vi "Get Map.vi"(8 "error in (no error)":errorcluster, 10 "URL":string) -> (0 "error out":errorcluster, 2 "Body":string)   [LabVIEW 2012]
doc: "Requests the given URL and returns the body of the request."
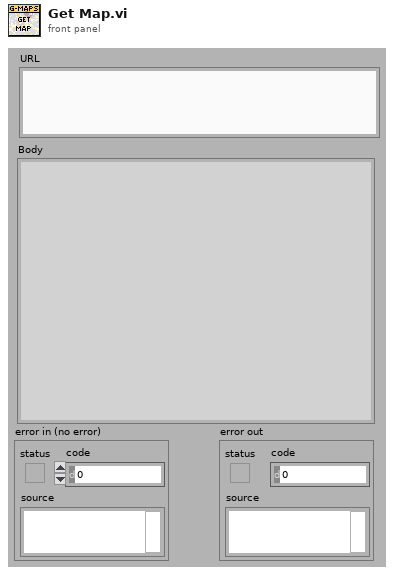
[diagram p1: front panel]
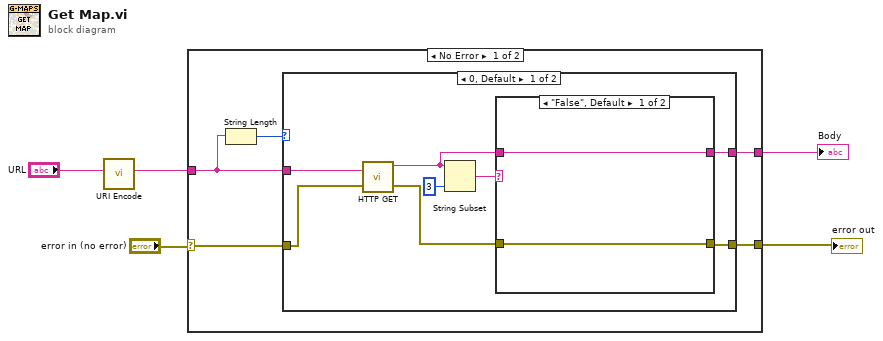
[diagram p0: block diagram]
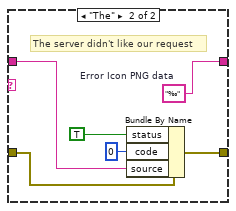
[diagram p2: hidden frame]
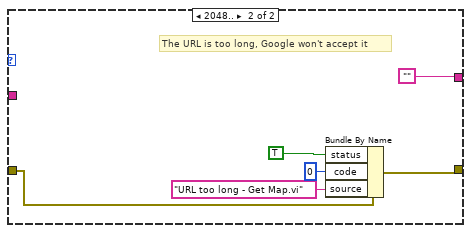
[diagram p3: hidden frame]
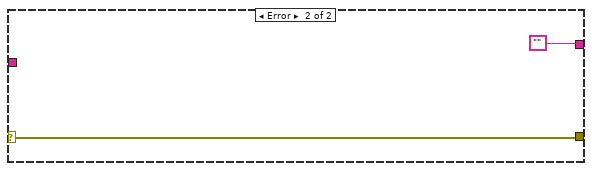
[diagram p4: hidden frame]
diagram:
  n1 = call "URI Encode.vi"("URL"="URL") -> ("URI out"=w1:string)  [unwired: 9 in, 1 out]
  n2 = case shown="No Error" "error in (no error)" {
    selector: "error in (no error)" -> [w8 w34]
    tunnel: w1 -> [w6 _]
    tunnel: [w10 w34] -> w5
    tunnel: [w9 ""] -> w4
    frame No Error {
      n3 = String Length(string=w6) -> (length=w7:i32)
      n4 = case shown="0, Default" w7 {
        tunnel: w6 -> [w18 _]
        tunnel: [w15 w29] -> w10
        tunnel: [w13 ""] -> w9
        tunnel: w8 -> [w11 w28]
        frame 0, Default {
          n5 = call "HTTP GET.vi"("error IO"=w11, "URI"=w18) -> ("error out"=w12:errorcluster, "body"=w14:string)
          n6 = String Subset(string=w14, length (rest)=3 ("length (rest)")) -> (substring=w16:string)  [unwired: 1 in]
          n7 = case shown="\"False\", Default" w16 {
            tunnel: w12 -> [w20 w25]
            tunnel: [w20 w26] -> w15
            tunnel: w14 -> [w19 w22]
            tunnel: [w19 w21] -> w13
            frame "False", Default {
            }
            frame "The" {
              w21 = "‰"  # Error Icon PNG data
              # "The server didn't like our request"
              n8 = Bundle By Name(cluster=w25, "status"=TRUE, "code"=0, "source"=w22) -> (w26:errorcluster)
            }
          }
        }
        frame 2048.. {
          # "The URL is too long, Google won't accept it"
          n9 = Bundle By Name(cluster=w28, "status"=TRUE, "code"=0, "source"="URL too long - Get Map.vi") -> (w29:errorcluster)
        }
      }
    }
    frame Error {
    }
  }
  "error out" <- w5
  "Body" <- w4
